vi "Close.vi"(8 "Error In":errorcluster, 11 "Hue Config":T1) -> (0 "Error Out":errorcluster)   [LabVIEW 2020, in "LMH-Hue.lvlib"]
uses:
  LMH-Hue.lvlib
  Private/Type Defs/Hue Ref.ctl
  <vilib>/httpClient/ClientHandle.ctl
  Private/Type Defs/Light Data.ctl
  <vilib>/httpClient/LabVIEWHTTPClient.lvlib
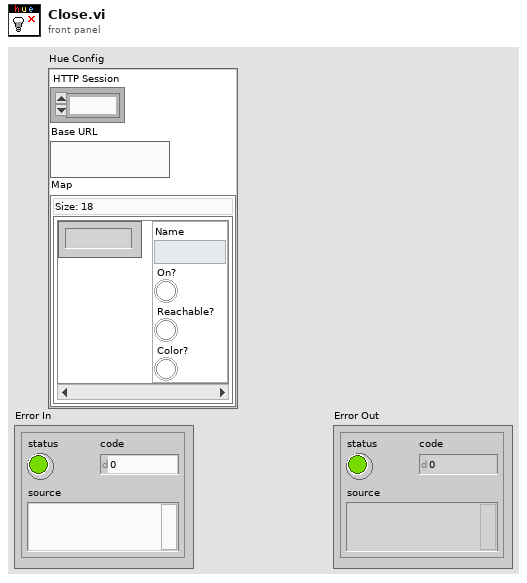
[diagram p1: front panel]
types:
  T1 = typedef "LMH-Hue.lvlib/Hue Ref.ctl" = cluster{"HTTP Session":T2, "Base URL":string, "Map":map{i32, T3}}
  T2 = typedef "LabVIEWHTTPClient.lvlib/ClientHandle.ctl" = refnum<k1>
  T3 = typedef "LMH-Hue.lvlib/Light Data.ctl" = cluster{"Name":string, "On?":bool, "Reachable?":bool, "Color?":bool}
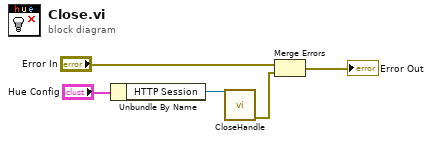
[diagram p0: block diagram]
diagram:
  n1 = Unbundle By Name("Hue Config") -> ("HTTP Session"=w4:T2)
  n2 = call <vilib>:"CloseHandle.vi"("client handle"=w4) -> ("error out"=w2:errorcluster)  [unwired: 14 in]
  n3 = Merge Errors("Error In", w2) -> (→"Error Out":errorcluster)
